vi "CernoxData-Auto-2009.vi"() -> ()   [LabVIEW 2009]
uses:
  <instrlib>/Lake Shore Cryotronics 370/Lake Shore Cryotronics 370.lvlib
panel:
  out "Estimated Temperature":dbl min=0.0 max=63200000.0 step=1e-05 format="%^.5e"
  out "Sensor 3 Resistance":dbl min=0.0 max=63200000.0 step=1e-05 format="%^.5e"
  out "Sensor 2 Resistance":dbl min=0.0 max=63200000.0 step=1e-05 format="%^.5e"
  out "Sensor 1 Resistance":dbl min=0.0 max=63200000.0 step=1e-05 format="%^.5e"
  out "Voltage Excitation in Use":i16
  out "Resistance vs Time":cluster{dbl[], dbl[]}[](graph)
  in  "File Path":path
  in  "Heater Range":u16(ring) items=["Off", "31.6 uA", "100 uA", "316 uA", "1.00 mA", "3.16 mA", "10.0 mA", "31.6 mA", "100 mA"]
  in  "Manual Output (0.000%)":dbl format="%#_13g"
  in  "(min)":dbl=5.0
  in  "(sec)":dbl
  in  "stop":bool
  # "Note that Sensor 1 is only valid between .3K and 325K. If you attempt to take a measurement outside of this range, this program will allow it, but those points aren't reliable for calibration of other thermometers!!! So switch to manual program if R1>=100k (T<.25 K)"
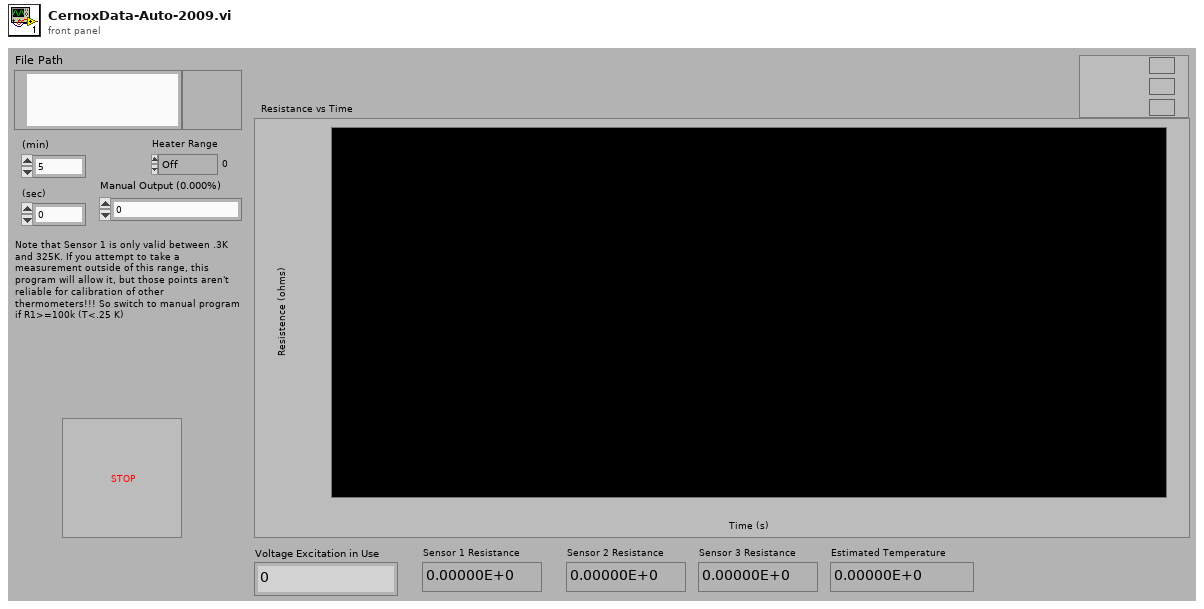
[diagram p1: front panel]
types:
  T1 = enum16{"open", "replace", "create", "open or create", "replace or create", "replace or create with confirmation"}
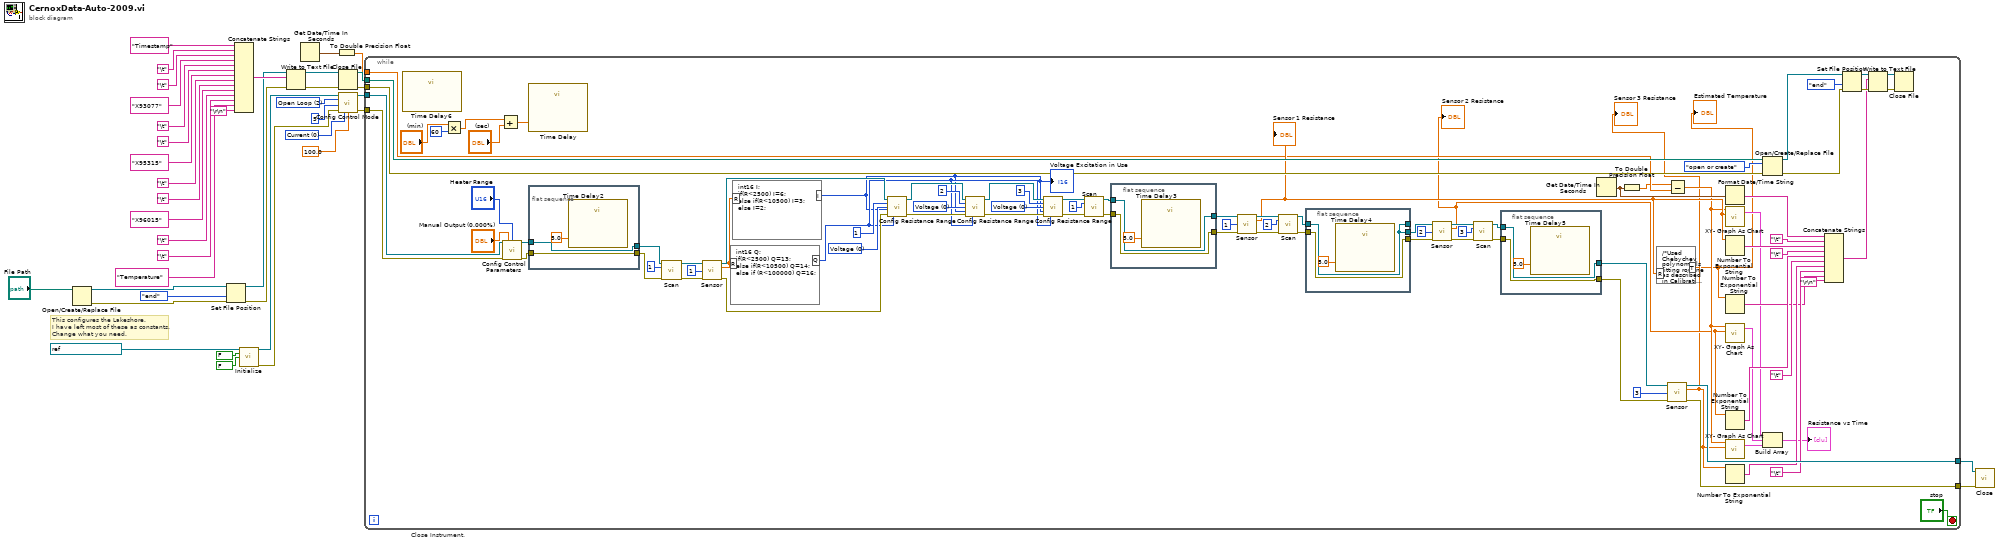
[diagram p0: block diagram]
diagram:
  w34 = u16 0 items=["Current", "Power"] ("Heater Output Display (0: Current)")
  w36 = u16 2 items=["Closed Loop PID", "Zone Tuning", "Open Loop", "Off"] ("Control Mode (0: Closed Loop PID)")
  # "This configures the Lakeshore.\nI have left most of these as constants.\nChange what you need."
  # "Close Instrument."
  n1 = Open/Create/Replace File(file path (use dialog)="File Path") -> (refnum out=w23:refnum<file>, error out=w27:errorcluster)  [unwired: 5 in, 1 out]
  n2 = Set File Position(refnum=w23, from (0:start)=enum16{"start", "end", "current"}."end", error in=w27) -> (refnum out=w22:refnum<file>, error out=w29:errorcluster)  [unwired: 1 in]
  n3 = Concatenate Strings("Timestamp" ("text"), "\t", "\t", "X93077" ("text"), "\t", "\t", "X95315" ("text"), "\t", "\t", "X96015" ("text"), "\t", "\t", "Temperature" ("text"), "\r\n") -> (w24:string)
  n4 = call <instrlib>:"Initialize.vi"("VISA resource name"=refnum<visa-resource-name> "GPIB0::11::INSTR" ("VISA Resource Name 2"), "ID Query (True)"=FALSE, "Reset (True)"=FALSE) -> ("VISA resource name out"=w38:refnum<visa-resource-name>, "error out"=w37:errorcluster)  [unwired: 11 in]
  n5 = Write to Text File(file (use dialog)=w22, text=w24, error in=w29) -> (refnum out=w21:refnum<file>, error out=w28:errorcluster)  [unwired: 1 in, 1 out]
  n6 = Get Date/Time In Seconds() -> (seconds since 1Jan1904=w2:timestamp)
  n7 = To Double Precision Float(number=w2) -> (double precision float=w1:dbl)
  n8 = Close File(refnum=w21, error in=w28) -> (path=w20:path, error out=w19:errorcluster)
  n9 = call <instrlib>:"Config Control Mode.vi"("VISA resource name"=w38, "Control Mode (0: Closed Loop PID)"=w36, "Channel (1)"=5, "error in (no error)"=w37, "Heater Output Display (0: Current)"=w34, "Heater Resistance (100.00)"=100.0) -> ("VISA resource name out"=w33:refnum<visa-resource-name>, "error out"=w32:errorcluster)  [unwired: 8 in]
  n10 = while {
    tunnel: w33 -> [w126]
    tunnel: w32 -> [w125]
    tunnel: [w112] -> w31
    tunnel: [w111] -> w30
    tunnel: w20 -> [w91]
    tunnel: w19 -> [w90]
    tunnel: w1 -> [w48]
    stop <- "stop" stop-if-true
    w85 = u16 0 items=["Voltage", "Current"] ("Excitation Mode (0: Voltage)")
    w87 = u16 0 items=["Voltage", "Current"] ("Excitation Mode (0: Voltage)")
    w89 = u16 0 items=["Voltage", "Current"] ("Excitation Mode (0: Voltage)")
    n11 = call "Time Delay6"() -> ()  [unwired: 11 in, 1 out]
    n12 = Multiply(x="(min)", y=60) -> (x*y=w130:dbl)
    n13 = Add(x=w130, y="(sec)") -> (x+y=w129:dbl)
    n14 = call <instrlib>:"Config Control Parameters.vi"("VISA resource name"=w126, "Manual Output (0.000%)"="Manual Output (0.000%)", "Heater Range (0: Off)"="Heater Range", "error in (no error)"=w125) -> ("VISA resource name out"=w75:refnum<visa-resource-name>, "error out"=w74:errorcluster)  [unwired: 10 in]
    n15 = call "Time Delay"("Delay Time (s)"=w129) -> ()  [unwired: 10 in, 1 out]
    n16 = flat-sequence {
      tunnel: w75 -> [w143]
      tunnel: w74 -> [w142]
      tunnel: [w143] -> w57
      tunnel: [w142] -> w56
      frame #0 {
        n17 = call "Time Delay2"("Delay Time (s)"=5.0) -> ()  [unwired: 10 in, 1 out]
      }
    }
    n18 = call <instrlib>:"Scan.vi"("VISA resource name"=w57, "Scan Channel (1)"=1, "error in (no error)"=w56) -> ("VISA resource name out"=w60:refnum<visa-resource-name>, "error out"=w59:errorcluster)  [unwired: 11 in]
    n19 = call <instrlib>:"Sensor.vi"("VISA resource name"=w60, "Channel (1)"=1, "error in (no error)"=w59) -> ("VISA resource name out"=w79:refnum<visa-resource-name>, "Resistance Reading"=w61:dbl, "error out"=w78:errorcluster)  [unwired: 8 in, 2 out]
    n20 = formula code="int16 Q;\nif(R<2500) Q=13;\nelse if(R<10500) Q=14;\nelse if (R<100000) Q=16;"("R"=w61) -> ("Q"=w45:i16)
    n21 = formula code="int16 I;\nif(R<2500) I=6;\nelse if(R<10500) I=3;\nelse I=2;"("R"=w61) -> ("I"=w44:i16)
    "Voltage Excitation in Use" <- w44
    n22 = call <instrlib>:"Config Resistance Range.vi"("VISA resource name"=w79, "Channel (1)"=1, "Excitation Mode (0: Voltage)"=w89, "Excitation Range (11: 632 mV / 316 nA)"=w44, "error in (no error)"=w78, "Resistance Range (21: 63.2 MOhm)"=w45) -> ("VISA resource name out"=w83:refnum<visa-resource-name>, "error out"=w82:errorcluster)  [unwired: 8 in]
    n23 = call <instrlib>:"Config Resistance Range.vi"("VISA resource name"=w83, "Channel (1)"=2, "Excitation Mode (0: Voltage)"=w87, "Excitation Range (11: 632 mV / 316 nA)"=w44, "error in (no error)"=w82, "Resistance Range (21: 63.2 MOhm)"=w45) -> ("VISA resource name out"=w81:refnum<visa-resource-name>, "error out"=w80:errorcluster)  [unwired: 8 in]
    n24 = call <instrlib>:"Config Resistance Range.vi"("VISA resource name"=w81, "Channel (1)"=3, "Excitation Mode (0: Voltage)"=w85, "Excitation Range (11: 632 mV / 316 nA)"=w44, "error in (no error)"=w80, "Resistance Range (21: 63.2 MOhm)"=w45) -> ("VISA resource name out"=w77:refnum<visa-resource-name>, "error out"=w76:errorcluster)  [unwired: 8 in]
    n25 = call <instrlib>:"Scan.vi"("VISA resource name"=w77, "Scan Channel (1)"=1, "error in (no error)"=w76) -> ("VISA resource name out"=w73:refnum<visa-resource-name>, "error out"=w72:errorcluster)  [unwired: 11 in]
    n26 = flat-sequence {
      tunnel: w73 -> [w140]
      tunnel: w72 -> [w139]
      tunnel: [w140] -> w71
      tunnel: [w139] -> w70
      frame #0 {
        n27 = call "Time Delay3"("Delay Time (s)"=5.0) -> ()  [unwired: 10 in, 1 out]
      }
    }
    n28 = call <instrlib>:"Sensor.vi"("VISA resource name"=w71, "Channel (1)"=1, "error in (no error)"=w70) -> ("VISA resource name out"=w121:refnum<visa-resource-name>, "Resistance Reading"=w50:dbl, "error out"=w120:errorcluster)  [unwired: 8 in, 2 out]
    "Sensor 1 Resistance" <- w50
    n29 = call <instrlib>:"Scan.vi"("VISA resource name"=w121, "Scan Channel (1)"=2, "error in (no error)"=w120) -> ("VISA resource name out"=w69:refnum<visa-resource-name>, "error out"=w68:errorcluster)  [unwired: 11 in]
    n30 = flat-sequence {
      tunnel: w69 -> [w136]
      tunnel: w68 -> [w137]
      tunnel: [w136] -> _
      tunnel: [w137] -> w66
      tunnel: [w136] -> w67
      frame #0 {
        n31 = call "Time Delay4"("Delay Time (s)"=5.0) -> ()  [unwired: 10 in, 1 out]
      }
    }
    n32 = call <instrlib>:"Sensor.vi"("VISA resource name"=w67, "Channel (1)"=2, "error in (no error)"=w66) -> ("VISA resource name out"=w117:refnum<visa-resource-name>, "Resistance Reading"=w43:dbl, "error out"=w115:errorcluster)  [unwired: 8 in, 2 out]
    "Sensor 2 Resistance" <- w43
    n33 = call <instrlib>:"Scan.vi"("VISA resource name"=w117, "Scan Channel (1)"=3, "error in (no error)"=w115) -> ("VISA resource name out"=w65:refnum<visa-resource-name>, "error out"=w64:errorcluster)  [unwired: 11 in]
    n34 = flat-sequence {
      tunnel: w65 -> [w134]
      tunnel: w64 -> [w133]
      tunnel: [w134] -> w63
      tunnel: [w133] -> w62
      frame #0 {
        n35 = call "Time Delay5"("Delay Time (s)"=5.0) -> ()  [unwired: 10 in, 1 out]
      }
    }
    n36 = Get Date/Time In Seconds() -> (seconds since 1Jan1904=w49:timestamp)
    n37 = To Double Precision Float(number=w49) -> (double precision float=w47:dbl)
    n38 = formula code="/*Used Chebychev polynomials fitting routine\nas described in Calibration Report Description \ndocument. For future use with other thermometer, \njust replace, in all the appropriate\nranges, the Chebychev coefficients (array 'A[i]'), \nthe lower and upper boundaries for Z (variables 'ZU' \nand 'ZL'), and the numberof polynomial terms or \nfit range (variable 'range'). This information is \nfound in the data file for the corresponding \nthermometer */\n\n/*Declare variables. Used same notation\nas Lakeshore Calibration Report Description*/\n\nfloat64 Z, ZL, ZU, X, T;\nfloat64 Tc[12], A[12];\nint range, i;\nZ=log(R);\n\n/*Fit range 1, for R between 967.9 and\n5.873e4*/\nif(R>967.9)\n{\nrange=9;\nZL= 2.9418494752;\nZU=5.02966374648;\nX=((Z-ZL)-(ZU-Z))/(ZU-ZL);\nA[0]=1.071498E+00;\nA[1]=-1.235482E+00;\nA[2]=6.21211E-01;\nA[3]=-2.81224E-01;\nA[4]=1.17945E-01;\nA[5]=-4.6423E-02;\nA[6]=1.7362E-02;\nA[7]=-6.436E-03;\nA[8]=1.773E-03;\nA[9]=-9.21E-04;\n\nTc[0]=1;\nTc[1]=X;\nT=A[0]+A[1]*X;\n\nfor(i=2; i<=range; i++)\n{\nTc[i]=2*X*Tc[i-1]-Tc[i-2];\nT=T+Tc[i]*A[i];\n}\n}\n\n/*Fit range 2, for R between 305.4 and\n967.9*/\nif(R>305.4 && R<=967.9)\n{\nrange=7;\nZL= 2.45731408995;\nZU= 3.03826253897;\nX=((Z-ZL)-(ZU-Z))/(ZU-ZL);\nA[0]=9.474723E+00;\nA[1]=-9.325816E+00;\nA[2]=3.081357E+00;\nA[3]=-7.35706E-01;\nA[4]=1.12233E-01;\nA[5]=-5.64E-04;\nA[6]=-5.762E-03;\nA[7]=1.5E-03;\n\nTc[0]=1;\nTc[1]=X;\nT=A[0]+A[1]*X;\n\nfor(i=2; i<=range; i++)\n{\nTc[i]=2*X*Tc[i-1]-Tc[i-2];\nT=T+Tc[i]*A[i];\n}\n}\n\n/*Fit range 3, for R between 128.8 and\n305.4*/\nif(R>128.8 && R<=305.4)\n{\nrange=7;\nZL= 2.06983873355;\nZU= 2.50740893552;\nX=((Z-ZL)-(ZU-Z))/(ZU-ZL);\nA[0]=5.5544531E+01;\nA[1]=-4.5102164E+01;\nA[2]=8.454989E+00;\nA[3]=-8.56752E-01;\nA[4]= 4.3477E-02;\nA[5]= 1.6502E-02;\nA[6]=-1.573E-03;\nA[7]=-2.692E-03;\n\nTc[0]=1;\nTc[1]=X;\nT=A[0]+A[1]*X;\n\nfor(i=2; i<=range; i++)\n{\nTc[i]=2*X*Tc[i-1]-Tc[i-2];\nT=T+Tc[i]*A[i];\n}\n}\n\n/*Fit range 4, for R between 55.45 and\n128.8*/\nif(R<=128.8)\n{\nrange=8;\nZL= 1.73925511291;\nZU= 2.13947962549;\nX=((Z-ZL)-(ZU-Z))/(ZU-ZL);\nA[0]=1.89660230E+02;\nA[1]=-1.20375552E+02;\nA[2]=1.7456024E+01;\nA[3]=-2.070901E00;\nA[4]= 3.76272E-01;\nA[5]=-6.009E-02;\nA[6]= 8.391E-03;\nA[7]=-1.551E-03;\nA[8]= 4.758E-03;\n\nTc[0]=1;\nTc[1]=X;\nT=A[0]+A[1]*X;\n\nfor(i=2; i<=range; i++)\n{\nTc[i]=2*X*Tc[i-1]-Tc[i-2];\nT=T+Tc[i]*A[i];\n}\n}"("R"=w50) -> ("T"=w41:dbl)
    "Estimated Temperature" <- w41
    n39 = call <instrlib>:"Sensor.vi"("VISA resource name"=w63, "Channel (1)"=3, "error in (no error)"=w62) -> ("VISA resource name out"=w112:refnum<visa-resource-name>, "Resistance Reading"=w42:dbl, "error out"=w111:errorcluster)  [unwired: 8 in, 2 out]
    "Sensor 3 Resistance" <- w42
    n40 = Subtract(x=w47, y=w48) -> (x-y=w46:dbl)
    n41 = Format Date/Time String(seconds (now)=w49) -> (date/time string=w93:string)  [unwired: 2 in]
    n42 = call <instrlib>:"XY- Graph As Chart.vi"("Y-Value"=w50, "X- Value"=w46) -> ("XY Graph"=w53:cluster{dbl[], dbl[]})  [unwired: 3 in]
    n43 = Number To Exponential String(number=w50) -> (E-format string=w97:string)  [unwired: 3 in]
    n44 = Number To Exponential String(number=w41) -> (E-format string=w95:string)  [unwired: 3 in]
    n45 = call <instrlib>:"XY- Graph As Chart.vi"("Y-Value"=w43, "X- Value"=w46) -> ("XY Graph"=w52:cluster{dbl[], dbl[]})  [unwired: 3 in]
    n46 = Number To Exponential String(number=w43) -> (E-format string=w101:string)  [unwired: 3 in]
    n47 = call <instrlib>:"XY- Graph As Chart.vi"("Y-Value"=w42, "X- Value"=w46) -> ("XY Graph"=w51:cluster{dbl[], dbl[]})  [unwired: 3 in]
    n48 = Number To Exponential String(number=w42) -> (E-format string=w98:string)  [unwired: 3 in]
    n49 = Open/Create/Replace File(file path (use dialog)=w91, error in=w90, operation (0:open)=T1."open or create") -> (refnum out=w106:refnum<file>, error out=w105:errorcluster)  [unwired: 3 in, 1 out]
    n50 = Build Array(w53, w52, w51) -> (→"Resistance vs Time":cluster{dbl[], dbl[]}[])
    n51 = Concatenate Strings(w93, "\t", w97, "\t", w101, "\t", w98, "\t", w95, "\r\n") -> (w102:string)
    n52 = Set File Position(refnum=w106, from (0:start)=enum16{"start", "end", "current"}."end", error in=w105) -> (refnum out=w110:refnum<file>, error out=w109:errorcluster)  [unwired: 1 in]
    n53 = Write to Text File(file (use dialog)=w110, text=w102, error in=w109) -> (refnum out=w108:refnum<file>, error out=w107:errorcluster)  [unwired: 1 in, 1 out]
    n54 = Close File(refnum=w108, error in=w107) -> ()  [unwired: 2 out]
  }
  n55 = call <instrlib>:"Close.vi"("VISA resource name"=w31, "error in (no error)"=w30) -> ()  [unwired: 13 in, 1 out]
